vi "Create.vi"(8 "error in (no error)":errorcluster, 10 "Input":string[](array[string])) -> (0 "error out":errorcluster, 3 "Map":refnum<class "Map.lvclass">)   [LabVIEW 2020, in "Map.lvclass"]
uses:
  Map.lvclass
  Map.lvclass/Map.ctl
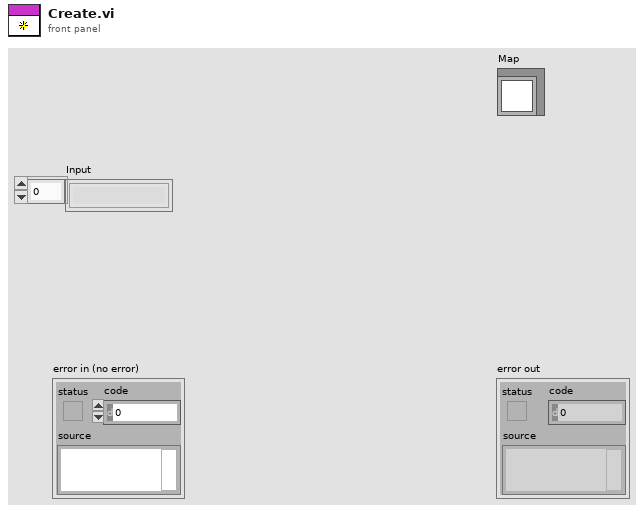
[diagram p1: front panel]
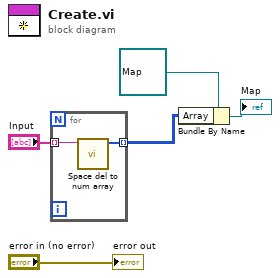
[diagram p0: block diagram]
diagram:
  n1 = for {
    tunnel: "Input" -> [w7] mode=indexing
    tunnel: [w6] -> w1 mode=indexing
    n2 = call "Space del to num array.vi"("Input in"=w7) -> ("Input out"=w6:u32[])  [unwired: 10 in]
  }
  n3 = Bundle By Name(cluster=refnum<class "Map.lvclass"> refnum ("Map"), "Array"=w1) -> (→"Map":refnum<class "Map.lvclass">)
  "error out" <- "error in (no error)"
